vi "yellowLabelDialog.vi"(11 "图片路径":string) -> ()   [LabVIEW 2011]
panel:
  out "pic":picture caption="新图片"
  out "bottom":i16
  out "right":i16
  out "top":i16
  out "left":i16
  out "缩放因子":sgl=1.0 format="%#.3g"
  in  "高":u32=720
  in  "长":u32=800
  in  "OK":bool
  # "请严格按照图示插线测试\n如果插反了，请先调换过来，然后点击“确定”继续测试"
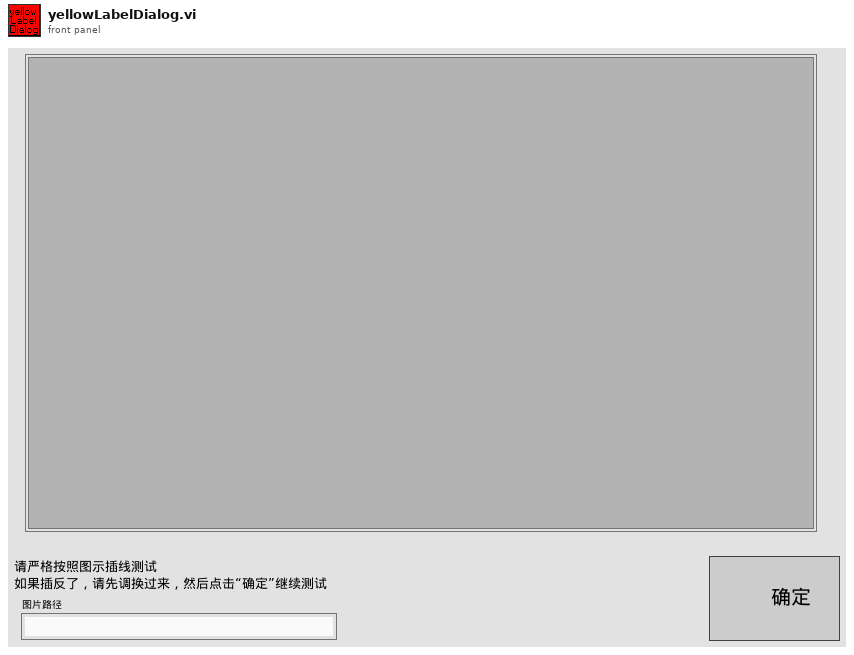
[diagram p1: front panel]
types:
  T1 = typedef "imagedata.ctl" = cluster{"image type":i32, "image depth":i32, "image":u8[], "mask":u8[], "colors":u32[], "Rectangle":cluster{"left":i16, "top":i16, "right":i16, "bottom":i16}}
  T2 = cluster{"left":i16, "top":i16, "right":i16, "bottom":i16}
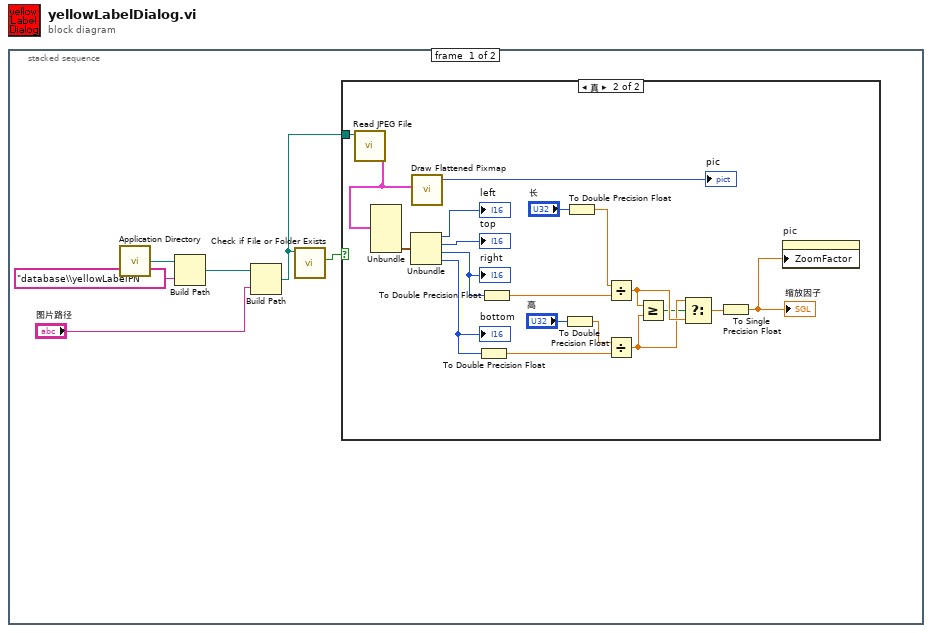
[diagram p0: block diagram]
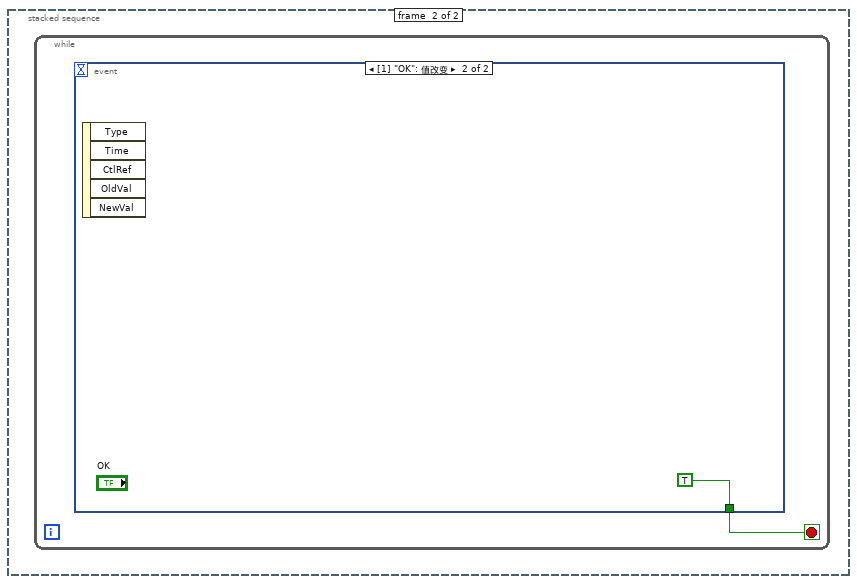
[diagram p3: hidden frame]
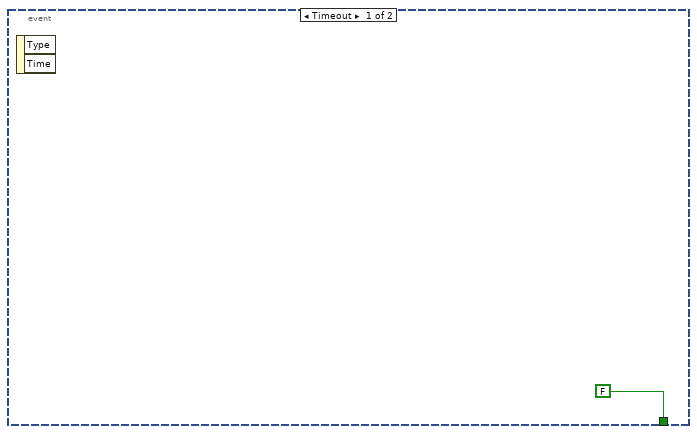
[diagram p4: hidden frame]
diagram:
  n1 = stacked-sequence {
    frame #0 {
      n2 = call <vilib>:"Application Directory.vi"() -> ("Application Directory"=w6:path)
      n3 = Build Path(base path=w6, name or relative path="database\\yellowLabelPN" ("名称或相对路径")) -> (appended path=w4:path)
      n4 = Build Path(base path=w4, name or relative path="图片路径") -> (appended path=w2:path)
      n5 = call <vilib>:"Check if File or Folder Exists.vi"("path"=w2) -> ("file or folder exists?"=w1:bool)  [unwired: 8 in, 2 out]
      n6 = case shown="真" w1 {
        tunnel: w2 -> [_ w7]
        frame False {
        }
        frame True {
          n7 = call <vilib>:"Read JPEG File.vi"("path to JPEG file"=w7) -> ("image data"=w11:T1)  [unwired: 8 in, 2 out]
          n8 = Unbundle(w11) -> ("Rectangle"=w20:T2)  [unwired: 5 out]
          n9 = Unbundle(w20) -> ("left"=→"left":i16, "top"=→"top":i16, "right"=w16:i16, "bottom"=w13:i16)
          "right" <- w16
          "bottom" <- w13
          n10 = call <vilib>:"Draw Flattened Pixmap.vi"("image data"=w11) -> ("new picture"=→"pic":picture)  [unwired: 8 in]
          n11 = To Double Precision Float(number=w13) -> (double precision float=w14:dbl)
          n12 = To Double Precision Float(number=w16) -> (double precision float=w18:dbl)
          n13 = To Double Precision Float(number="高") -> (double precision float=w15:dbl)
          n14 = To Double Precision Float(number="长") -> (double precision float=w17:dbl)
          n15 = Divide(x=w17, y=w18) -> (x/y=w25:dbl)
          n16 = Divide(x=w15, y=w14) -> (x/y=w24:dbl)
          n17 = Greater Or Equal?(x=w25, y=w24) -> (x >= y?=w23:bool)
          n18 = Select(t=w24, s=w23, f=w25) -> (s? t:f=w12:dbl)
          n19 = To Single Precision Float(number=w12) -> (single precision float=w8:sgl)
          "缩放因子" <- w8
          n20 = property on="pic" class="Pict"("ZoomFactor"=w8) -> ()  [unwired: 2 in, 2 out]
        }
      }
    }
    frame #1 {
      n21 = while {
        stop <- w26 stop-if-true
        n22 = event shown="[1] \"OK\": 值改变" {
          selector: _ -> [_ _]
          dyn-events: _ -> [_ _]
          timeout: _ -> [_ _]
          tunnel: [FALSE TRUE] -> w26
          event Timeout {
            n23 = event-data() -> ()  [unwired: 1 in, 2 out]
          }
          event "OK": Value Change {
            n24 = event-data() -> ()  [unwired: 1 in, 5 out]
          }
        }
      }
    }
  }
